vi "Move Direction.vi"(10 "Direction":T1, 11 "cluster in":cluster{"Row":i32, "Col":i32}) -> (3 "cluster out":cluster{"Row":i32, "Col":i32})   [LabVIEW 2023]
uses:
  ENUM_Direction.ctl
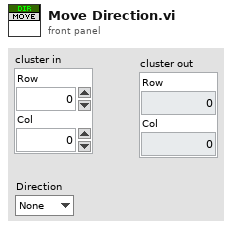
[diagram p1: front panel]
types:
  T1 = typedef "ENUM_Direction.ctl" = enum16{"None", "N", "S", "E", "W"}
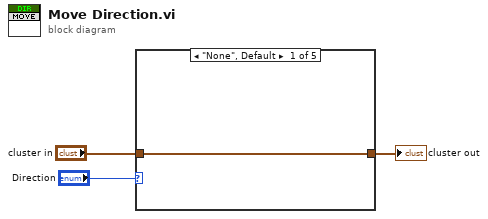
[diagram p0: block diagram]
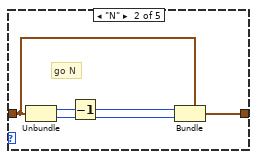
[diagram p2: hidden frame]
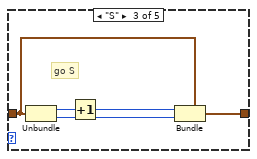
[diagram p3: hidden frame]
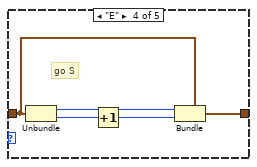
[diagram p4: hidden frame]
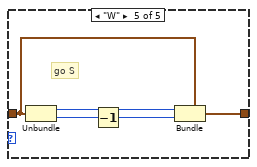
[diagram p5: hidden frame]
diagram:
  n1 = case shown="\"None\", Default" "Direction" {
    tunnel: "cluster in" -> [w4 w9 w14 w19 w24]
    tunnel: [w4 w8 w13 w18 w23] -> w2
    frame "None", Default {
    }
    frame "N" {
      # "go N"
      n2 = Unbundle(w9) -> ("Row"=w7:i32, "Col"=w5:i32)
      n3 = Decrement(x=w7) -> (x-1=w6:i32)
      n4 = Bundle(cluster=w9, "Row"=w6, "Col"=w5) -> (w8:cluster{"Row":i32, "Col":i32})
    }
    frame "S" {
      # "go S"
      n5 = Unbundle(w14) -> ("Row"=w12:i32, "Col"=w10:i32)
      n6 = Increment(x=w12) -> (x+1=w11:i32)
      n7 = Bundle(cluster=w14, "Row"=w11, "Col"=w10) -> (w13:cluster{"Row":i32, "Col":i32})
    }
    frame "E" {
      # "go S"
      n8 = Unbundle(w19) -> ("Row"=w16:i32, "Col"=w17:i32)
      n9 = Increment(x=w17) -> (x+1=w15:i32)
      n10 = Bundle(cluster=w19, "Row"=w16, "Col"=w15) -> (w18:cluster{"Row":i32, "Col":i32})
    }
    frame "W" {
      # "go S"
      n11 = Unbundle(w24) -> ("Row"=w21:i32, "Col"=w22:i32)
      n12 = Decrement(x=w22) -> (x-1=w20:i32)
      n13 = Bundle(cluster=w24, "Row"=w21, "Col"=w20) -> (w23:cluster{"Row":i32, "Col":i32})
    }
  }
  "cluster out" <- w2
